vi "Make Commands Absolute.vi"(8 "error in (no error)":errorcluster, 11 "Tool Path in":refnum<class "Tool Path.lvclass">) -> (0 "error out":errorcluster, 3 "Tool Path out":refnum<class "Tool Path.lvclass">)   [LabVIEW 2019, in "Tool Path.lvclass"]
uses:
  Tool Path.lvclass
  Parse/ParsePaths/Path.lvclass/Path.ctl
  Parse/PathCommands/PathCommands.lvclass
  Parse/ParsePaths/Path.lvclass
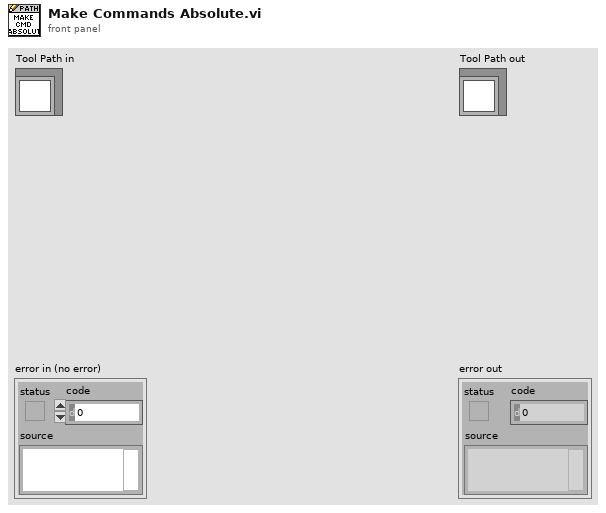
[diagram p1: front panel]
types:
  T1 = typedef "PathCommands.lvclass/Point.ctl" = cluster{"X":dbl, "Y":dbl}
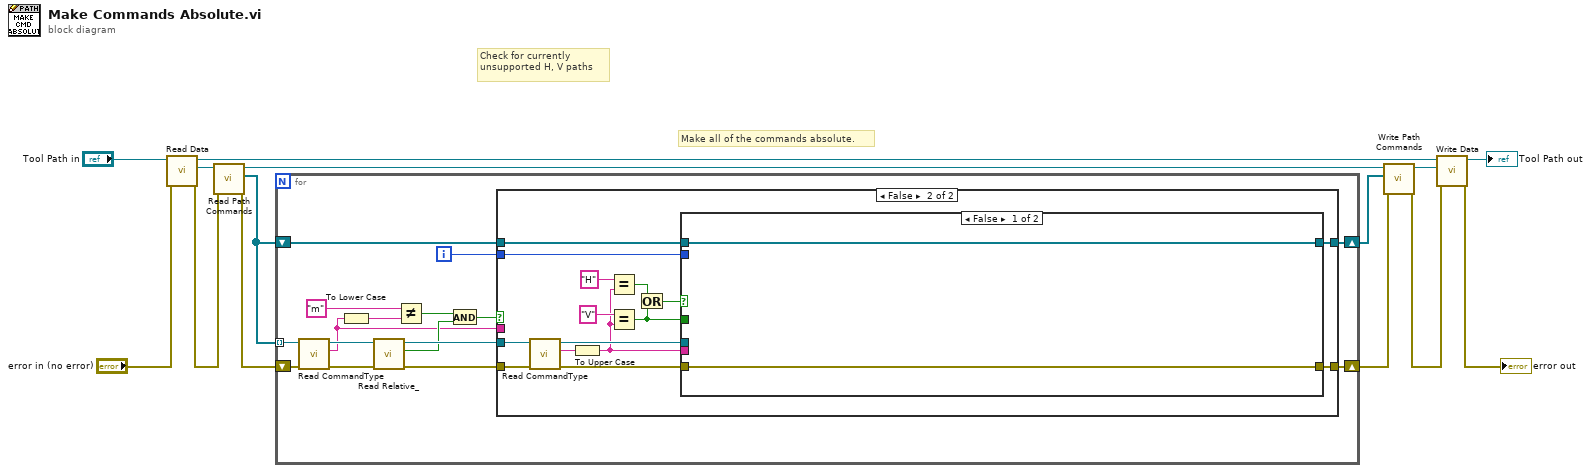
[diagram p0: block diagram]
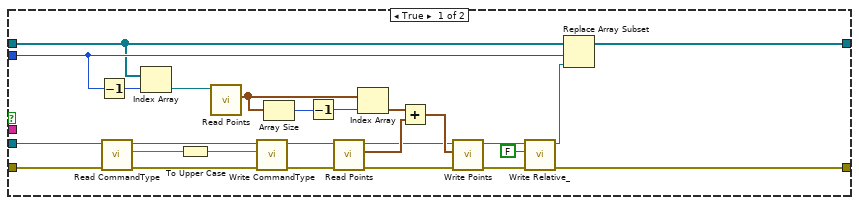
[diagram p2: hidden frame]
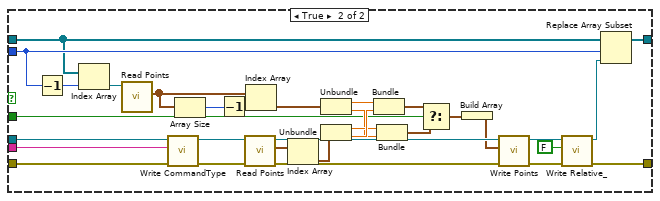
[diagram p3: hidden frame]
diagram:
  # "Check for currently unsupported H, V paths"
  # "Make all of the commands absolute."
  n1 = call-dynamic "Read Data.vi"("error in (no error)"="error in (no error)", "Tool Path in"="Tool Path in") -> ("error out"=w3:errorcluster, "Path.lvclass"=w8:refnum<class "Path.lvclass">, "Tool Path out"=w7:refnum<class "Tool Path.lvclass">)  [unwired: 7 in]
  n2 = call "Read Path Commands.vi"("error in (no error)"=w3, "Path in"=w8) -> ("error out"=w13:errorcluster, "Path Commands"=w14:refnum<class "PathCommands.lvclass">[], "Path out"=w12:refnum<class "Path.lvclass">)  [unwired: 7 in]
  n3 = for {
    tunnel: w14 -> [w26] mode=indexing
    shift-right: [w21] -> w11
    shift-left: w13 -> [w20]
    shift-right: [w19] -> w10
    shift-left: w14 -> [w29]
    i -> [w28]
    n4 = call-dynamic "Read CommandType.vi"("error in (no error)"=w20, "PathCommands in"=w26) -> ("error out"=w23:errorcluster, "CommandType"=w15:string, "PathCommands out"=w27:refnum<class "PathCommands.lvclass">)  [unwired: 7 in]
    n5 = To Lower Case(string=w15) -> (all lower case string=w18:string)
    n6 = call-dynamic "Read Relative_.vi"("error in (no error)"=w23, "PathCommands in"=w27) -> ("error out"=w22:errorcluster, "Relative?"=w24:bool, "PathCommands out"=w30:refnum<class "PathCommands.lvclass">)  [unwired: 7 in]
    n7 = Not Equal?(x="m", y=w18) -> (x != y?=w25:bool)
    n8 = And(x=w25, y=w24) -> (x .and. y?=w16:bool)
    n9 = case shown="False" w16 {
      tunnel: w30 -> [w42 w70]
      tunnel: w29 -> [w31 w63]
      tunnel: w28 -> [w32 w64]
      tunnel: w22 -> [w37 w67]
      tunnel: [w35 w66] -> w21
      tunnel: [w33 w65] -> w19
      tunnel: w15 -> [_ _]
      frame True {
        n10 = Decrement(x=w32) -> (x-1=w56:i32)
        n11 = call-dynamic "Read CommandType.vi"("error in (no error)"=w37, "PathCommands in"=w42) -> ("error out"=w39:errorcluster, "CommandType"=w41:string, "PathCommands out"=w44:refnum<class "PathCommands.lvclass">)  [unwired: 7 in]
        n12 = Index Array(array=w31, index=w56) -> (element=w55:refnum<class "PathCommands.lvclass">)
        n13 = To Upper Case(1:w41) -> (0:w40:string)
        n14 = call-dynamic "Read Points.vi"("PathCommands in"=w55) -> ("Points"=w53:T1[])  [unwired: 8 in, 2 out]
        n15 = call-dynamic "Write CommandType.vi"("error in (no error)"=w39, "CommandType"=w40, "PathCommands in"=w44) -> ("error out"=w38:errorcluster, "PathCommands out"=w43:refnum<class "PathCommands.lvclass">)  [unwired: 7 in]
        n16 = Array Size(array=w53) -> (size(s)=w54:i32)
        n17 = Decrement(x=w54) -> (x-1=w52:i32)
        n18 = call-dynamic "Read Points.vi"("error in (no error)"=w38, "PathCommands in"=w43) -> ("error out"=w36:errorcluster, "Points"=w50:T1[], "PathCommands out"=w45:refnum<class "PathCommands.lvclass">)  [unwired: 7 in]
        n19 = Index Array(array=w53, index=w52) -> (element=w51:T1)
        n20 = Add(x=w51, y=w50) -> (x+y=w49:T1[])
        n21 = call-dynamic "Write Points.vi"("error in (no error)"=w36, "Points"=w49, "PathCommands in"=w45) -> ("error out"=w46:errorcluster, "PathCommands out"=w48:refnum<class "PathCommands.lvclass">)  [unwired: 7 in]
        n22 = call-dynamic "Write Relative_.vi"("error in (no error)"=w46, "Relative?"=FALSE, "PathCommands in"=w48) -> ("error out"=w35:errorcluster, "PathCommands out"=w34:refnum<class "PathCommands.lvclass">)  [unwired: 7 in]
        n23 = Replace Array Subset(array=w31, new element=w34, index=w32) -> (w33:refnum<class "PathCommands.lvclass">[])
      }
      frame False {
        n24 = call-dynamic "Read CommandType.vi"("error in (no error)"=w67, "PathCommands in"=w70) -> ("error out"=w68:errorcluster, "CommandType"=w69:string, "PathCommands out"=w71:refnum<class "PathCommands.lvclass">)  [unwired: 7 in]
        n25 = To Upper Case(1:w69) -> (0:w60:string)
        n26 = Equal?(x="H", y=w60) -> (x = y?=w59:bool)
        n27 = Equal?(x="V", y=w60) -> (x = y?=w57:bool)
        n28 = Or(x=w59, y=w57) -> (x .or. y?=w58:bool)
        n29 = case shown="False" w58 {
          tunnel: w71 -> [_ w96]
          tunnel: w60 -> [_ w94]
          tunnel: w68 -> [w72 w93]
          tunnel: [w72 w90] -> w66
          tunnel: [w73 w88] -> w65
          tunnel: w64 -> [_ w87]
          tunnel: w63 -> [w73 w86]
          tunnel: w57 -> [_ w76]
          frame False {
          }
          frame True {
            n30 = Decrement(x=w87) -> (x-1=w105:i32)
            n31 = Index Array(array=w86, index=w105) -> (element=w104:refnum<class "PathCommands.lvclass">)
            n32 = call-dynamic "Read Points.vi"("PathCommands in"=w104) -> ("Points"=w102:T1[])  [unwired: 8 in, 2 out]
            n33 = call-dynamic "Write CommandType.vi"("error in (no error)"=w93, "CommandType"=w94, "PathCommands in"=w96) -> ("error out"=w92:errorcluster, "PathCommands out"=w95:refnum<class "PathCommands.lvclass">)  [unwired: 7 in]
            n34 = Array Size(array=w102) -> (size(s)=w103:i32)
            n35 = Decrement(x=w103) -> (x-1=w101:i32)
            n36 = call-dynamic "Read Points.vi"("error in (no error)"=w92, "PathCommands in"=w95) -> ("error out"=w91:errorcluster, "Points"=w84:T1[], "PathCommands out"=w97:refnum<class "PathCommands.lvclass">)  [unwired: 7 in]
            n37 = Index Array(array=w102, index=w101) -> (element=w85:T1)
            n38 = Index Array(array=w84) -> (element=w83:T1)  [unwired: 1 in]
            n39 = Unbundle(w85) -> ("X"=w82:dbl, "Y"=w79:dbl)
            n40 = Unbundle(w83) -> ("X"=w80:dbl, "Y"=w81:dbl)
            n41 = Bundle("X"=w82, "Y"=w81) -> (w78:cluster{"X":dbl, "Y":dbl})  [unwired: 1 in]
            n42 = Bundle("X"=w80, "Y"=w79) -> (w77:cluster{"X":dbl, "Y":dbl})  [unwired: 1 in]
            n43 = Select(t=w78, s=w76, f=w77) -> (s? t:f=w75:cluster{"X":dbl, "Y":dbl})
            n44 = Build Array(w75) -> (w74:cluster{"X":dbl, "Y":dbl}[])
            n45 = call-dynamic "Write Points.vi"("error in (no error)"=w91, "Points"=w74, "PathCommands in"=w97) -> ("error out"=w98:errorcluster, "PathCommands out"=w100:refnum<class "PathCommands.lvclass">)  [unwired: 7 in]
            n46 = call-dynamic "Write Relative_.vi"("error in (no error)"=w98, "Relative?"=FALSE, "PathCommands in"=w100) -> ("error out"=w90:errorcluster, "PathCommands out"=w89:refnum<class "PathCommands.lvclass">)  [unwired: 7 in]
            n47 = Replace Array Subset(array=w86, new element=w89, index=w87) -> (w88:refnum<class "PathCommands.lvclass">[])
          }
        }
      }
    }
  }
  n48 = call "Write Path Commands.vi"("error in (no error)"=w11, "Path Commands"=w10, "Path in"=w12) -> ("error out"=w2:errorcluster, "Path out"=w9:refnum<class "Path.lvclass">)  [unwired: 7 in]
  n49 = call-dynamic "Write Data.vi"("error in (no error)"=w2, "Path.lvclass"=w9, "Tool Path in"=w7) -> ("error out"=→"error out":errorcluster, "Tool Path out"=→"Tool Path out":refnum<class "Tool Path.lvclass">)  [unwired: 7 in]
